vi "Enum from Value.vi"(10 "Value":i32) -> (2 "Enumeration":T1)   [LabVIEW 2020, in "Enum Template.lvlib"]
uses:
  Enum Template.lvlib
  Enumeration.ctl
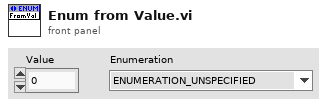
[diagram p1: front panel]
types:
  T1 = typedef "Enum Template.lvlib/Enumeration.ctl" = enum16{"ENUMERATION_UNSPECIFIED"}
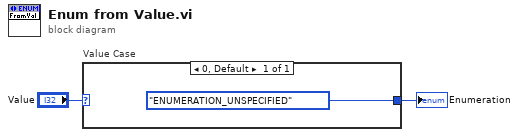
[diagram p0: block diagram]
diagram:
  n1 = case "Value Case" shown="0, Default" "Value" {
    tunnel: [Enumeration."ENUMERATION_UNSPECIFIED" ("Enumeration")] -> w1
    frame 0, Default {
    }
  }
  "Enumeration" <- w1
